vi "Send Commands(SubVI).vi"(10 "Number of Particles after":i32, 11 "Cluster":T1) -> ()   [LabVIEW 2014]
uses:
  Global.vi
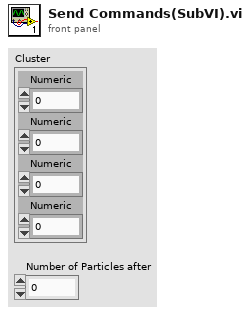
[diagram p1: front panel]
types:
  T1 = cluster{"Numeric":dbl, "Numeric":dbl, "Numeric":dbl, "Numeric":dbl}
  T2 = typedef "Control cluster.ctl" = cluster{"Roll":sgl, "Pitch":sgl, "Vertical Speed":sgl, "Yaw Speed":sgl}
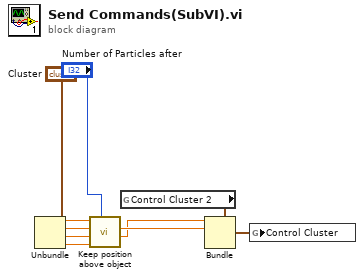
[diagram p0: block diagram]
diagram:
  n1 = Unbundle("Cluster") -> ("Numeric"=w4:dbl, "Numeric"=w5:dbl, "Numeric"=w6:dbl, "Numeric"=w7:dbl)
  n2 = call "Keep position above object.vi"("nr of particles"="Number of Particles after", "bottom"=w7, "right"=w6, "top"=w5, "left"=w4) -> ("Roll"=w2:dbl, "Pitch"=w3:dbl)  [unwired: 4 in, 1 out]
  n3 = global read "Global.vi" "Control Cluster 2"() -> (w10:T2)
  n4 = Bundle(cluster=w10, "Roll"=w2, "Pitch"=w3) -> (w1:T2)  [unwired: 2 in]
  n5 = global write "Global.vi" "Control Cluster"(w1) -> ()
